vi "Log Error to File.vi"(8 "error in (no error)":errorcluster) -> ()   [LabVIEW 2020, in "Error Handler.lvclass"]
uses:
  Error Handler.lvclass
  Support/Utilities.lvlib
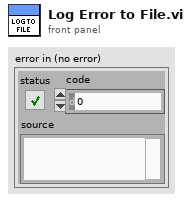
[diagram p1: front panel]
types:
  T1 = enum16{"open", "replace", "create", "open or create", "replace or create", "replace or create with confirmation"}
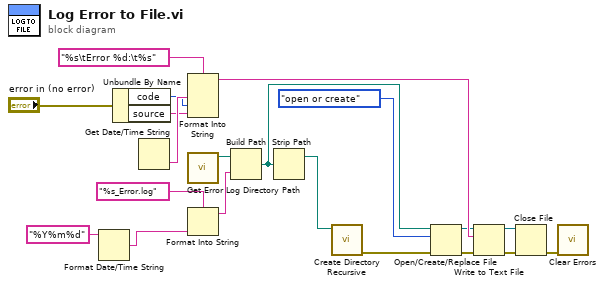
[diagram p0: block diagram]
diagram:
  n1 = Format Date/Time String(time format string (%c)="%Y%m%d") -> (date/time string=w1:string)  [unwired: 2 in]
  n2 = Unbundle By Name("error in (no error)") -> ("code"=w17:i32, "source"=w18:string)
  n3 = Get Date/Time String() -> (time string=w19:string)  [unwired: 3 in, 1 out]
  n4 = Format Into String(format string="%s\tError %d:\t%s", w19, w17, w18) -> (resulting string=w20:string)  [unwired: 2 in, 1 out]
  n5 = call "Get Error Log Directory Path.vi"() -> ("Error Log Path"=w7:path)  [unwired: 11 in]
  n6 = Format Into String(format string="%s_Error.log", w1) -> (resulting string=w8:string)  [unwired: 2 in, 1 out]
  n7 = Build Path(base path=w7, name or relative path=w8) -> (appended path=w9:path)
  n8 = Strip Path(path=w9) -> (stripped path=w4:path)  [unwired: 1 out]
  n9 = call <vilib>:"Create Directory Recursive.vi"("directory"=w4) -> ("error out"=w3:errorcluster)  [unwired: 4 in, 2 out]
  n10 = Open/Create/Replace File(file path (use dialog)=w9, error in=w3, operation (0:open)=T1."open or create") -> (refnum out=w10:refnum<file>, error out=w11:errorcluster)  [unwired: 3 in, 1 out]
  n11 = Write to Text File(file (use dialog)=w10, text=w20, error in=w11) -> (refnum out=w12:refnum<file>, error out=w13:errorcluster)  [unwired: 1 in, 1 out]
  n12 = Close File(refnum=w12, error in=w13) -> (error out=w14:errorcluster)  [unwired: 1 out]
  n13 = call <vilib>:"Clear Errors.vi"("error in (no error)"=w14) -> ()  [unwired: 5 in, 2 out]
